vi "spdLib Test.vi"() -> ()   [LabVIEW 2018]
uses:
  hidSPDLibForLabView.lvlib
panel:
  out "Ready":bool[](array[boolean])
  out "Diod T":T1(graph)
  out "Heatsink T":T1(graph)
  in  "Stop":bool
  out "error out":errorcluster
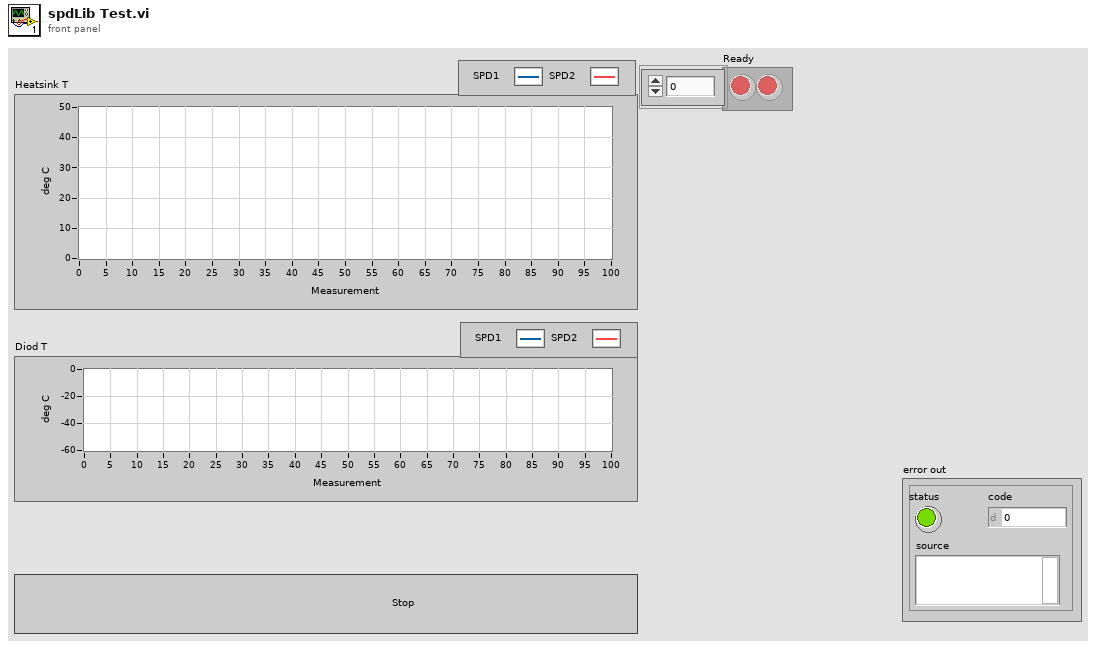
[diagram p1: front panel]
types:
  T1 = cluster{"Heatsink Tempratures[0]":sgl, "Heatsink Tempratures[1]":sgl}
  T2 = cluster{"Heatsink Tempratures[0]":sgl, "Heatsink Tempratures[1]":sgl}[]
  T3 = typedef "hidSPDLibForLabView.lvlib/hidSPD HidDevInfo.ctl" = cluster{"name":string, "path":string}
  T4 = typedef "hidSPDLibForLabView.lvlib/hidSPD Device Session.ctl" = cluster{"spdDevicePointer":u64}
  T5 = typedef "hidSPDLibForLabView.lvlib/hidSPD Simple Report.ctl" = cluster{"Heatsink Temprature":sgl, "Diod Temprature":sgl, "TEC-voltage":sgl, "Diod Bias":sgl, "RF Power":sgl, "Thermal used":sgl, "hv bias used":sgl, "hv code used":u16, "strobe code used":u16, "SPD number":u8, "SPD ready":u8}
  T6 = cluster{"Diod Tempratures[0]":sgl, "Diod Tempratures[1]":sgl}
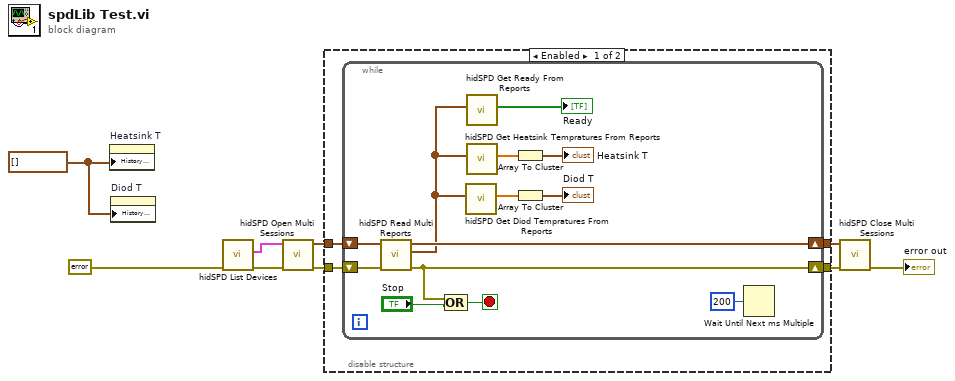
[diagram p0: block diagram]
diagram:
  w1 = T2 [] ("History Data")
  n1 = property on="Heatsink T" class="WFChart (strict)"("History Data"=w1) -> ()  [unwired: 2 in, 2 out]
  n2 = property on="Diod T" class="WFChart (strict)"("History Data"=w1) -> ()  [unwired: 2 in, 2 out]
  n3 = call "hidSPD List Devices.vi"("error in (no error)"=errorcluster {"status"=FALSE, "code"=0, "source"=""}) -> ("error out"=w7:errorcluster, "devices list"=w8:T3[])  [unwired: 9 in]
  n4 = call "hidSPD Open Multi Sessions.vi"("error in (no error)"=w7, "devices list"=w8) -> ("error out"=w4:errorcluster, "spdDevSessions out"=w5:T4[])  [unwired: 8 in]
  n5 = disable-structure shown="Enabled" {
    disable-tunnel: w5 -> [w13 w28]
    disable-tunnel: w4 -> [w12 w27]
    disable-tunnel: [w11 w28] -> w3
    disable-tunnel: [w10 w27] -> w2
    frame Enabled {
      n6 = while {
        shift-right: [w24] -> w11
        shift-left: w13 -> [w26]
        shift-right: [w22] -> w10
        shift-left: w12 -> [w25]
        stop <- w21 stop-if-true
        n7 = call "hidSPD Read Multi Reports.vi"("error in (no error)"=w25, "spdDevSessions in"=w26) -> ("error out"=w22:errorcluster, "spd Reports"=w15:T5[], "spdDevSessions out"=w24:T4[])  [unwired: 7 in]
        n8 = Compound Arithmetic op=OR(w22, "Stop") -> (w21:bool)
        n9 = call "hidSPD Get Diod Tempratures From Reports.vi"("spd Reports in"=w15) -> ("Diod Tempratures"=w19:sgl[])  [unwired: 10 in]
        n10 = call "hidSPD Get Ready From Reports.vi"("spd Reports in"=w15) -> ("Ready"=→"Ready":bool[])  [unwired: 10 in]
        n11 = call "hidSPD Get Heatsink Tempratures From Reports.vi"("spd Reports in"=w15) -> ("Heatsink Tempratures"=w17:sgl[])  [unwired: 10 in]
        n12 = Array To Cluster(array=w17) -> (cluster=→"Heatsink T":T1)
        n13 = Array To Cluster(array=w19) -> (cluster=→"Diod T":T6)
        n14 = Wait Until Next ms Multiple(millisecond multiple=u32 200) -> ()  [unwired: 1 out]
      }
    }
    frame Disabled {
    }
  }
  n15 = call "hidSPD Close Multi Sessions.vi"("error in (no error)"=w2, "spdDevSessions out"=w3) -> ("error out"=→"error out":errorcluster)  [unwired: 9 in]
